vi "New TCP.vi"(7 "library path":path=path "libmodbus.so.5", 8 "error in (no error)":errorcluster, 10 "port":i32=502, 11 "ip address":string) -> (0 "error out":errorcluster, 3 "modbus out":refnum<class "libmodbus.lvclass">)   [LabVIEW 2017, in "libmodbus.lvlib" / "libmodbus.lvclass"]
doc: "create a libmodbus context for TCP/IPv4"
uses:
  libmodbus.lvclass
  libmodbus.lvclass/libmodbus.ctl
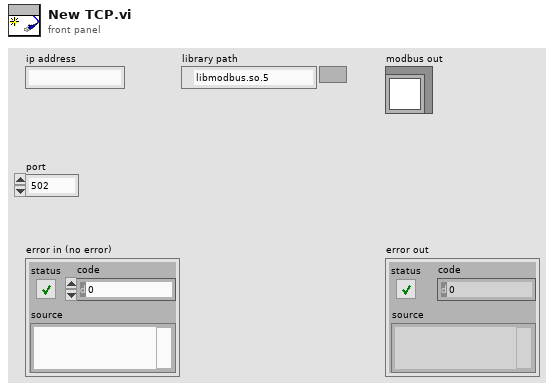
[diagram p1: front panel]
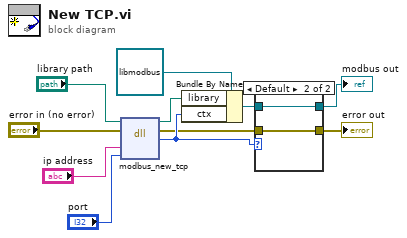
[diagram p0: block diagram]
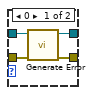
[diagram p2: hidden frame]
diagram:
  n1 = dll-call lib="?" fn="modbus_new_tcp"(path in="library path", error in="error in (no error)", "ip"="ip address", "port"="port") -> (path out=w7:path, error out=w4:errorcluster, "modbus_t"=w5:i64)  [unwired: 3 in]
  n2 = Bundle By Name(cluster=refnum<class "libmodbus.lvclass"> refnum ("modbus out"), "library"=w7, "ctx"=w5) -> (w2:refnum<class "libmodbus.lvclass">)
  n3 = case shown="Default" w5 {
    tunnel: w4 -> [w13 w17]
    tunnel: [w12 w17] -> w3
    tunnel: w2 -> [w15 w16]
    tunnel: [w14 w16] -> w1
    frame 0 {
      n4 = call "Generate Error.vi"("error in (no error)"=w13, "modbus in"=w15) -> ("error out"=w12:errorcluster, "modbus out"=w14:refnum<class "libmodbus.lvclass">)  [unwired: 8 in]
    }
    frame Default {
    }
  }
  "error out" <- w3
  "modbus out" <- w1
